vi "RLwithTD.vi"() -> ()   [LabVIEW 2019]
uses:
  <vilib>/Platform/TimedLoop/XDataNode/timing_clust.ctl
  <vilib>/Platform/TimedLoop/XDataNode/nitl_modes.ctl
  <vilib>/Platform/TimedLoop/XDataNode/wakeup.ctl
  <vilib>/Simulation/Shared/_Datatypes/SIM SISO Transfer Function.ctl
  <vilib>/myRIO/Instrument Drivers/Onboard IO/AI/typedefs/AI Reference.ctl
  <vilib>/myRIO/Common/Instrument Driver Framework/Utilities/typedefs/myRIO Generic Hardware Reference.ctl
  <vilib>/myRIO/Common/Instrument Driver Framework/Utilities/typedefs/Hardware Version Enum.ctl
  <vilib>/myRIO/Common/Instrument Driver Framework/Utilities/typedefs/myRIO v1.0 Reference.ctl
  <vilib>/myRIO/Common/Instrument Driver Framework/Utilities/typedefs/Generic FPGA Reference.ctl
  <vilib>/myRIO/Common/Instrument Driver Framework/myRIO v1.0/AI/typedefs/AI Channels List.ctl
  <vilib>/myRIO/Common/Instrument Driver Framework/myRIO v1.0/AI/typedefs/AI Channels Enum.ctl
  <vilib>/myRIO/Common/Instrument Driver Framework/Utilities/typedefs/Analog Scaling Constants List.ctl
  <vilib>/myRIO/Common/Instrument Driver Framework/Utilities/typedefs/Analog Scaling Constants.ctl
  <vilib>/userDefined/High Color/nirio_resource_hc.ctl
  <vilib>/Simulation/Shared/_Datatypes/SIM MIMO State Space.ctl
  <vilib>/myRIO/Instrument Drivers/Onboard IO/AO/typedefs/AO Reference.ctl
  <vilib>/myRIO/Common/Instrument Driver Framework/myRIO v1.0/AO/typedefs/AO Channels List.ctl
  <vilib>/myRIO/Common/Instrument Driver Framework/myRIO v1.0/AO/typedefs/AO Channels Enum.ctl
  <vilib>/myRIO/Common/Instrument Driver Framework/Utilities/vis/Is FPGA Ref Available.vi
  <vilib>/myRIO/Common/Instrument Driver Framework/myRIO v1.0/AI/vis/myRIO v1.1 Open AI.vi
  <vilib>/myRIO/Instrument Drivers/Onboard IO/AI/vis/Read.vi
  <vilib>/Simulation/DiscreteLinear/Implementation/NILVSim Discrete Transfer Function Direct.llb/SIM Discrete Transfer Function Diagram (SISO).vi
  <vilib>/Simulation/DiscreteLinear/Implementation/NILVSim Discrete State Space Direct.llb/SIM Discrete State Space Direct Diagram (SISO).vi
  <vilib>/myRIO/Common/Instrument Driver Framework/myRIO v1.0/AO/vis/myRIO v1.1 Open AO.vi
  <vilib>/myRIO/Instrument Drivers/Onboard IO/AO/vis/Write.vi
  <vilib>/myRIO/Common/Instrument Driver Framework/Utilities/vis/Validate Channels.vi
  <vilib>/myRIO/Common/Instrument Driver Framework/myRIO v1.0/AI/vis/myRIO v1.0 Reserve AI.vi
  <vilib>/Simulation/ContinuousLinear/Implementation/Shared/SIM Transfer Function Support.llb/SIM TransferFunction Normalize to Buffer.vi
  <vilib>/Simulation/DiscreteLinear/Implementation/Shared/SIM Init Discrete States.vi
  <vilib>/Simulation/DiscreteLinear/Implementation/NILVSim Discrete Transfer Function Direct.llb/SIM Transfer Function Direct core (SISO).vi
  <vilib>/Simulation/DiscreteLinear/Implementation/NILVSim Discrete State Space Direct.llb/NILVSim Discrete State Space Direct Diagram Core (SISO).vi
  <vilib>/myRIO/Common/Instrument Driver Framework/myRIO v1.0/AO/vis/myRIO v1.0 Reserve AO.vi
  <vilib>/myRIO/Common/Instrument Driver Framework/myRIO v1.0/AI/vis/myRIO v1.0 Build MUX Configuration AI.vi
  <vilib>/myRIO/Common/Instrument Driver Framework/myRIO v1.0/Resource Manager/vis/myRIO v1.0 Reserve Channel List.vi
  <vilib>/Simulation/ContinuousLinear/Implementation/Shared/SIM Transfer Function Support.llb/SIM TransferFunction Normalize.vi
  <vilib>/myRIO/Common/Instrument Driver Framework/myRIO v1.0/AO/vis/myRIO v1.0 Build MUX Configuration AO.vi
  <vilib>/myRIO/Common/Instrument Driver Framework/myRIO v1.0/Resource Manager/vis/myRIO v1.0 Reserve Channel.vi
  <vilib>/myRIO/Common/Instrument Driver Framework/myRIO v1.0/Resource Manager/vis/myRIO v1.0 Unreserve Channel.vi
  <vilib>/Simulation/Implementation/Shared/SIM Polynomials.llb/SIM Remove Zero Coefficients (DBL).vi
  <vilib>/myRIO/Common/Instrument Driver Framework/myRIO v1.0/Resource Manager/vis/myRIO v1.0 Build Mutex Name.vi
  <vilib>/Simulation/Implementation/Shared/SIM Polynomials.llb/SIM Divide Polynomials (DBL).vi
  <vilib>/Simulation/Implementation/Shared/SIM BuildSimErr.vi
  <vilib>/Utility/VariantDataType/GetNumericInfo.vi
  <vilib>/Utility/error.llb/Error Cluster From Error Code.vi
  <vilib>/myRIO/Common/Instrument Driver Framework/myRIO v1.0/myRIO v1.1 Open.vi
  <vilib>/myRIO/Common/Instrument Driver Framework/myRIO v1.0/AI/vis/myRIO v1.0 Get Scaling Constants AI.vi
  <vilib>/myRIO/Common/Instrument Driver Framework/Utilities/vis/IO Manager.vi
  <vilib>/myRIO/Common/Instrument Driver Framework/Utilities/vis/Configuration Manager.vi
  <vilib>/myRIO/Common/Instrument Driver Framework/myRIO v1.0/myRIO v1.0 Close.vi
  <vilib>/myRIO/Common/Instrument Driver Framework/myRIO v1.0/AI/vis/myRIO v1.0 Read AI.vi
  <vilib>/myRIO/Common/Instrument Driver Framework/myRIO v1.0/AO/vis/myRIO v1.0 Get Scaling Constants AO.vi
  <vilib>/myRIO/Common/Instrument Driver Framework/myRIO v1.0/AO/vis/myRIO v1.0 Write AO.vi
  <vilib>/platform/TimedLoop/XDataNode/XDataNode.xnode
  <vilib>/Simulation/Implementation/XNodeFramework/SimXNode/SimX.xnode
  <vilib>/myRIO/Express VI/Onboard IO/AI/AI Express VI.xnode
  <vilib>/myRIO/Instrument Drivers/Onboard IO/AI/vis/myRIO AI Open.xnode
  <vilib>/myRIO/Express VI/Onboard IO/AO/AO Express VI.xnode
  <vilib>/myRIO/Instrument Drivers/Onboard IO/AO/vis/myRIO AO Open.xnode
  <vilib>/Platform/TimedLoop/XDataNode/XDNodeRunTimeDep.lvlib
  <vilib>/myRIO/Instrument Drivers/Onboard IO/AI/AI.lvlib
  <vilib>/myRIO/Instrument Drivers/Onboard IO/AO/AO.lvlib
  <vilib>/ptbypt/NI_PtbyPt.lvlib
panel:
  out "element":dbl
  in  "Chtter off":bool=TRUE
  in  "psi":dbl=1.0
  in  "Ks":dbl=10.0
  in  "b":dbl=5.0
  in  "hm":dbl=0.01
  in  "Amp step":dbl format="%0.2f"
  in  "D":dbl=16.7
  in  "P":dbl=4689.8
  in  "stopNoise":bool=TRUE
  in  "gain_noise":dbl=0.2
  out "uniform white noise":dbl(graph)=-0.0799803013769669
  in  "AmpWhitehNoise":dbl=1.0 format="%0.2f"
  out "Iteration Duration":i64(graph)=243
  in  "Max FRF current 0-1000mA":dbl=4.0
  in  "Stop FRF":bool=TRUE
  in  "esc":bool
  out "scope":T1(graph)
  out "Current Output EM":dbl(graph)
  in  "Stop EM + FRF":bool=TRUE
  out "left[V]":dbl=-0.0
  out "right[V]":dbl=-0.0
  out "um":dbl=442.3828578
  # "mA"
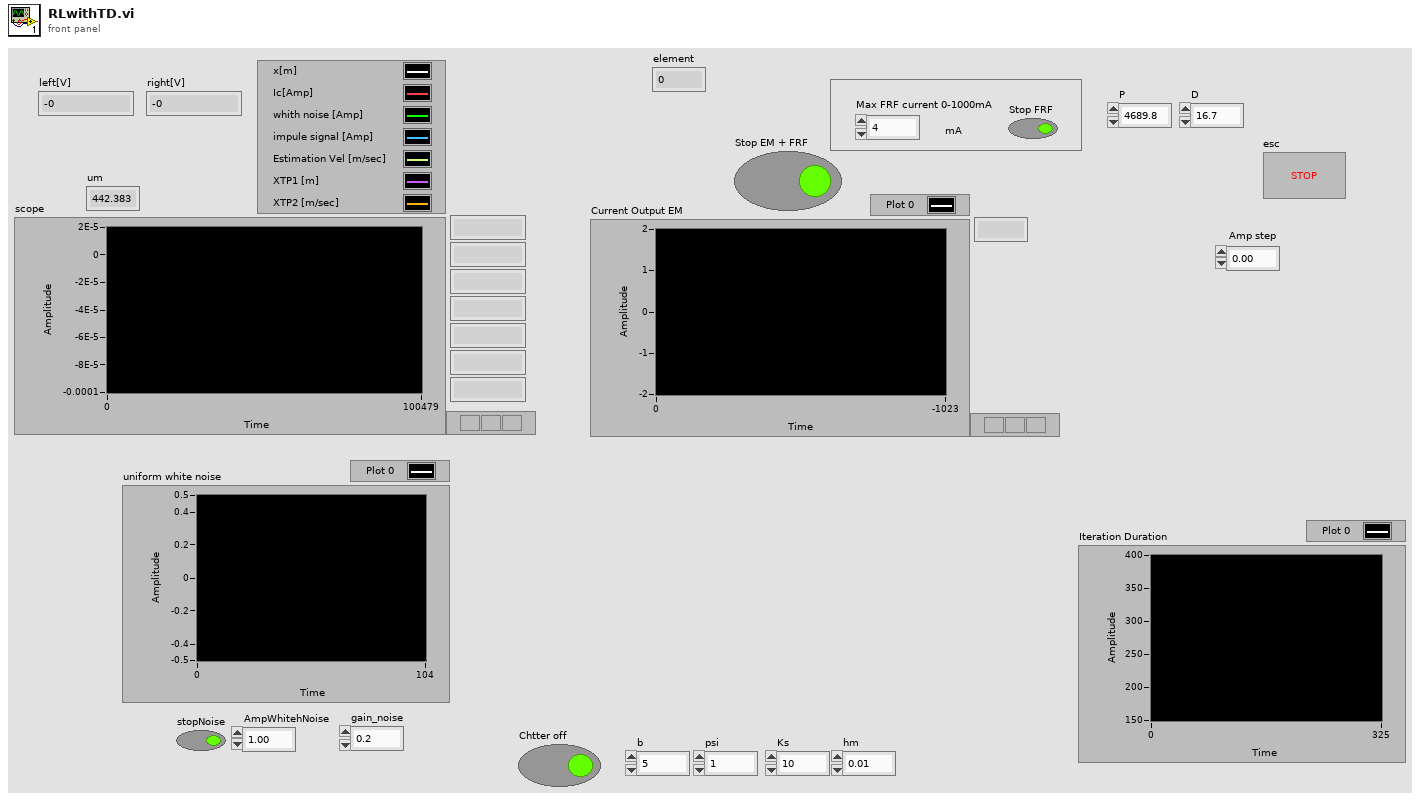
[diagram p1: front panel]
types:
  T1 = cluster{dbl, dbl, dbl, "output y(k)":dbl, dbl, "Numeric":dbl, "Numeric":dbl}
  T2 = typedef "XDNodeRunTimeDep.lvlib/timing_clust.ctl" = cluster{"Expected End [f-1]":u64, "Actual End [f-1]":u64, "Finished Late? [f-1]":bool, "Expected End [i-1]":u64, "Actual End [i-1]":u64, "Finished Late? [i-1]":bool, "Expected Start [i]":u64, "Actual Start [i]":u64, "Expected Start [f]":u64, "Actual Start [f]":u64, "Source Name":string, "Structure Name":string, "Period":i64, "Deadline":i64, "Offset":i64, "Start":i64, "Priority":i32, "Timeout":i32, "Mode":T3, "Wakeup Reason":T4, "Error":errorcluster, "Source Type":string, "Secondary Source Type":string, "Global End Time":u64, "Global Start Time":u64, "Frame Duration":u64, "Iteration Duration":u64, "Assigned CPU":i32, "I/O Scan Engine Mode":u32}
  T3 = typedef "XDNodeRunTimeDep.lvlib/nitl_modes.ctl" = enum32{"No Change", "Process missed periods, maintain original phase", "Discard missed periods, maintain original phase", "Process missed periods, ignore original phase", "Discard missed periods, ignore original phase"}
  T4 = typedef "XDNodeRunTimeDep.lvlib/wakeup.ctl" = enum32{"Normal", "Aborted", "Asynchronous wakeup", "Timing source error", "Timed loop error", "Timeout"}
  T5 = typedef "SIM SISO Transfer Function.ctl" = cluster{"Numerator":dbl[], "Denominator":dbl[]}
  T6 = typedef "SIM MIMO State Space.ctl" = cluster{"A":dbl[][], "B":dbl[][], "C":dbl[][], "D":dbl[][]}
  T7 = typedef "AO.lvlib/AO Reference.ctl" = cluster{"myRIO Reference":T8, "AO Channel List":T12, "AO Scaling Constant List":T14}
  T8 = typedef "myRIO Generic Hardware Reference.ctl" = cluster{"myRIO Model":T9, "myRIO Hardware Reference":T10}
  T9 = typedef "Hardware Version Enum.ctl" = enum16{"Unknown", "myRIO-1900", "myRIO-1950", "roboRIO", "NI ELVIS RIO CM", "ELVIS III"}
  T10 = typedef "myRIO v1.0 Reference.ctl" = cluster{"Generic FPGA Reference":T11, "Allow multiple opens":bool}
  T11 = typedef "Generic FPGA Reference.ctl" = refnum<k20>
  T12 = typedef "AO Channels List.ctl" = T13[]
  T13 = typedef "AO Channels Enum.ctl" = enum16{"Not Connected", "AudioOut/Left", "AudioOut/Right", "C/AO0", "C/AO1", "A/AO0", "A/AO1", "B/AO0", "B/AO1"}
  T14 = typedef "Analog Scaling Constants List.ctl" = T15[]
  T15 = typedef "Analog Scaling Constants.ctl" = cluster{"LSB Weight (Volts)":dbl, "Offset (Volts)":dbl, "Signed?":bool}
  T16 = typedef "nirio_resource_hc.ctl" = tag
  T17 = typedef "AI.lvlib/AI Reference.ctl" = cluster{"myRIO Reference":T8, "AI Channels List":T18, "AI Scaling Constants List":T14}
  T18 = typedef "AI Channels List.ctl" = T19[]
  T19 = typedef "AI Channels Enum.ctl" = enum16{"Not Connected", "AudioIn/Left", "AudioIn/Right", "C/AI0", "C/AI1", "A/AI0", "A/AI1", "A/AI2", "A/AI3", "A/AI4", "A/AI5", "A/AI6", "A/AI7", "B/AI0", "B/AI1", "B/AI2", "B/AI3", "B/AI4", "B/AI5", "B/AI6", "B/AI7", "AI/AI0", "AI/AI1", "AI/AI2", "AI/AI3", "A/AI0 (DIFF)", "A/AI1 (DIFF)", "A/AI2 (DIFF)", "A/AI3 (DIFF)", "B/AI0 (DIFF)", "B/AI1 (DIFF)", "B/AI2 (DIFF)", "B/AI3 (DIFF)"}
  T20 = cluster{dbl, dbl, dbl, dbl, "output y(k)":dbl, "Numeric":dbl, "Numeric":dbl}
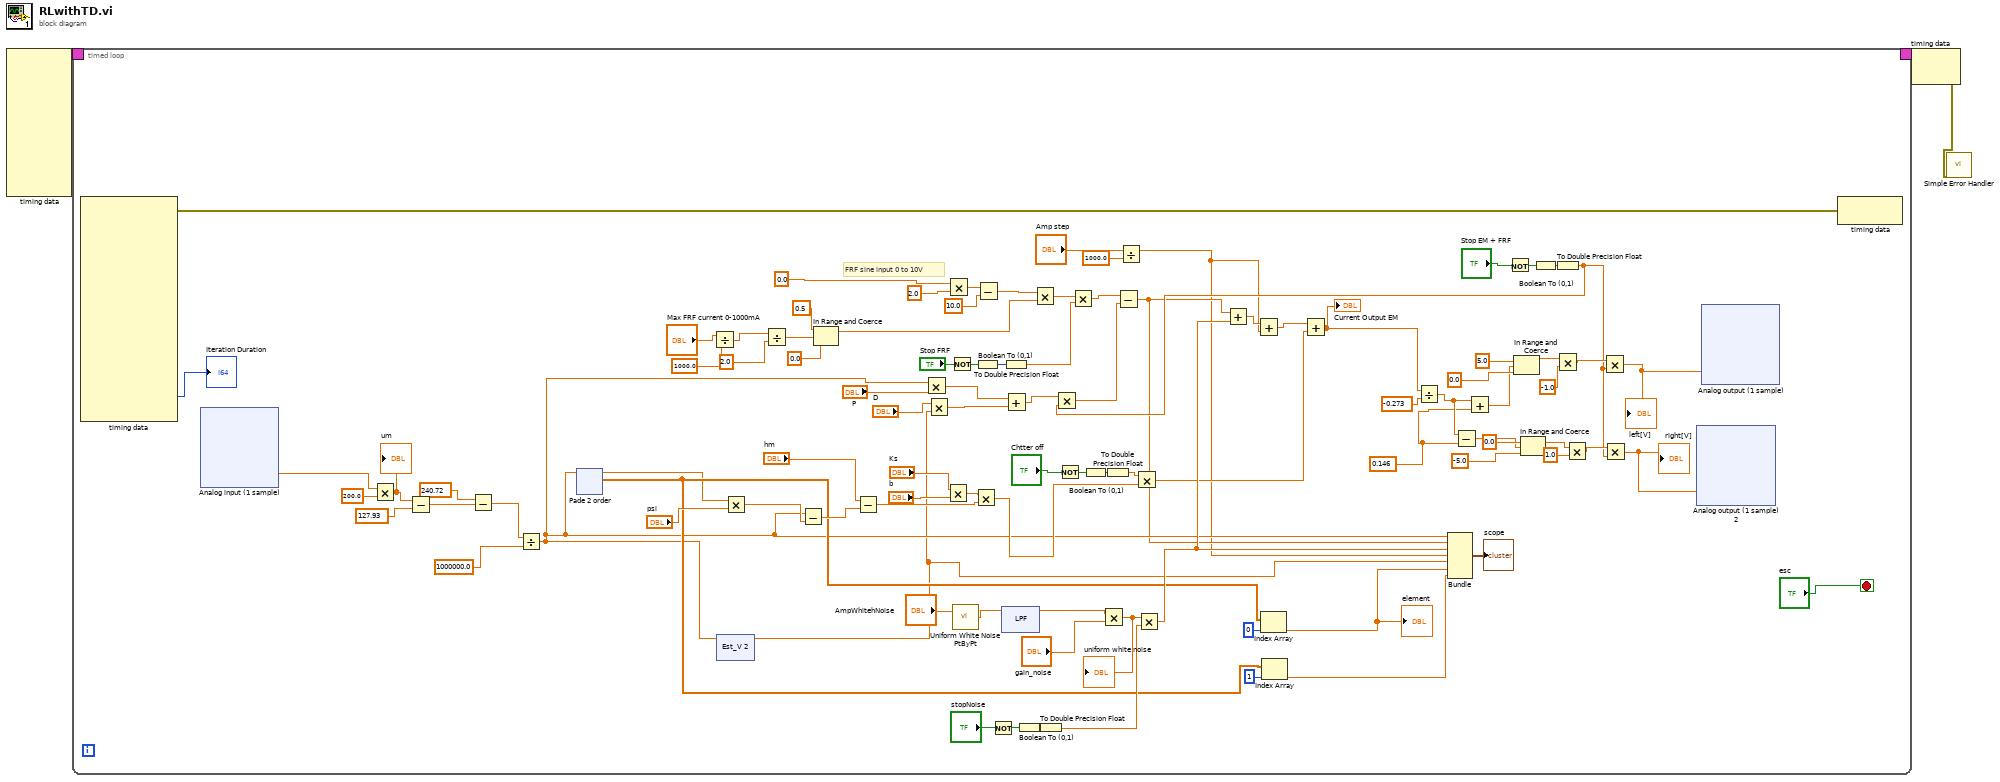
[diagram p0: block diagram]
diagram:
  n1 = node-c288() -> (w3:T2)  [unwired: 10 in]
  n2 = timed-loop {
    timing: w3 -> [_]
    timing-out: [_] -> w2
    stop <- "esc" stop-if-true
    w60 = 0.146 ("y")
    # "FRF sine input 0 to 10V"
    n3 = node-c288() -> (w100:errorcluster, →"Iteration Duration":i64)  [unwired: 1 in, 15 out]
    n4 = xnode "Analog input (1 sample)"() -> ("C/AI1 (AI1)"=w57:dbl)  [unwired: 1 in, 1 out]
    n5 = Multiply(x=w57, y=200.0) -> (x*y=w98:dbl)
    "um" <- w98
    n6 = Subtract(x=w98, y=127.93) -> (x-y=w97:dbl)
    n7 = Subtract(x=240.72, y=w97) -> (x-y=w42:dbl)
    n8 = Divide(x=w42, y=1000000.0) -> (x/y=w8:dbl)
    n9 = xnode "Pade 2 order"("input u(k)"=w8) -> ("state x(k+1)"=w12:dbl[], "output y(k)"=w9:dbl)  [unwired: 2 in, 2 out]
    n10 = Divide(x="Max FRF current 0-1000mA", y=1000.0) -> (x/y=w67:dbl)
    n11 = xnode "Est_V 2"("input u(k)"=w8) -> ("output y(k)"=w7:dbl)  [unwired: 2 in, 1 out]
    n12 = Multiply(x=w9, y="psi") -> (x*y=w18:dbl)
    n13 = Divide(x=w67, y=2.0) -> (x/y=w71:dbl)
    n14 = Subtract(x=w8, y=w18) -> (x-y=w17:dbl)
    n15 = In Range and Coerce(upper limit=0.5, x=w71, lower limit=0.0) -> (coerced(x)=w68:dbl)  [unwired: 1 out]
    n16 = Subtract(x="hm", y=w17) -> (x-y=w32:dbl)
    n17 = Multiply(x=w8, y="P") -> (x*y=w41:dbl)
    n18 = Multiply(x="D", y=w7) -> (x*y=w40:dbl)
    n19 = Multiply(x="Ks", y="b") -> (x*y=w33:dbl)
    n20 = Multiply(x=0.0, y=2.0) -> (x*y=w76:dbl)
    n21 = Not(x="Stop FRF") -> (.not. x?=w80:bool)
    n22 = call <vilib>:"Uniform White Noise PtByPt.vi"("amplitude"="AmpWhitehNoise") -> ("uniform white noise"=w51:dbl)  [unwired: 2 in]
    n23 = Multiply(x=w33, y=w32) -> (x*y=w24:dbl)
    n24 = Boolean To (0,1)(Boolean=w80) -> (0, 1=w79:i16)
    n25 = Subtract(x=w76, y=10.0) -> (x-y=w73:dbl)
    n26 = Not(x="stopNoise") -> (.not. x?=w49:bool)
    n27 = xnode "LPF"("input u(k)"=w51) -> ("output y(k)"=w48:dbl)  [unwired: 2 in, 1 out]
    n28 = To Double Precision Float(number=w79) -> (double precision float=w78:dbl)
    n29 = Add(x=w41, y=w40) -> (x+y=w34:dbl)
    n30 = Boolean To (0,1)(Boolean=w49) -> (0, 1=w50:i16)
    n31 = Multiply(x=w73, y=w68) -> (x*y=w74:dbl)
    n32 = To Double Precision Float(number=w50) -> (double precision float=w45:dbl)
    n33 = Not(x="Chtter off") -> (.not. x?=w26:bool)
    n34 = Multiply(x=w74, y=w78) -> (x*y=w82:dbl)
    n35 = Boolean To (0,1)(Boolean=w26) -> (0, 1=w27:i16)
    n36 = Multiply(x=w48, y="gain_noise") -> (x*y=w44:dbl)
    "uniform white noise" <- w44
    n37 = To Double Precision Float(number=w27) -> (double precision float=w25:dbl)
    n38 = Divide(x="Amp step", y=1000.0) -> (x/y=w5:dbl)
    n39 = Multiply(x=w25, y=w24) -> (x*y=w23:dbl)
    n40 = Multiply(x=w44, y=w45) -> (x*y=w43:dbl)
    n41 = Index Array(array=w12, index=0 ("index (row)")) -> (element=w15:dbl)
    "element" <- w15
    n42 = Index Array(array=w12, index=1) -> (element=w14:dbl)
    n43 = Not(x="Stop EM + FRF") -> (.not. x?=w85:bool)
    n44 = Boolean To (0,1)(Boolean=w85) -> (0, 1=w87:i16)
    n45 = To Double Precision Float(number=w87) -> (double precision float=w35:dbl)
    n46 = Multiply(x=w34, y=w35) -> (x*y=w36:dbl)
    n47 = Subtract(x=w82, y=w36) -> (x-y=w6:dbl)
    n48 = Add(x=w6, y=w43) -> (x+y=w39:dbl)
    n49 = Add(x=w39, y=w5) -> (x+y=w19:dbl)
    n50 = Add(x=w19, y=w23) -> (x+y=w20:dbl)
    "Current Output EM" <- w20
    n51 = Divide(x=w20, y=-0.273) -> (x/y=w61:dbl)
    n52 = Bundle(w8, w6, w43, w5, "output y(k)"=w7, "Numeric"=w15, "Numeric"=w14) -> (→"scope":T20)  [unwired: 1 in]
    n53 = Subtract(x=w61, y=w60) -> (x-y=w62:dbl)
    n54 = Add(x=w61, y=w60) -> (x+y=w63:dbl)
    n55 = In Range and Coerce(upper limit=5.0 ("x"), x=w63, lower limit=0.0) -> (coerced(x)=w54:dbl)  [unwired: 1 out]
    n56 = In Range and Coerce(upper limit=0.0 ("x"), x=w62, lower limit=-5.0) -> (coerced(x)=w90:dbl)  [unwired: 1 out]
    n57 = Multiply(x=w54, y=-1.0) -> (x*y=w59:dbl)
    n58 = Multiply(x=w90, y=1.0) -> (x*y=w58:dbl)
    n59 = Multiply(x=w59, y=w35) -> (x*y=w56:dbl)
    "left[V]" <- w56
    n60 = Multiply(x=w58, y=w35) -> (x*y=w55:dbl)
    "right[V]" <- w55
    n61 = xnode "Analog output (1 sample) 2"("C/AO1 (AO1)"=w55) -> ()  [unwired: 1 in, 1 out]
    n62 = xnode "Analog output (1 sample)"("C/AO0 (AO0)"=w56) -> ()  [unwired: 1 in, 1 out]
    n63 = node-c288(w100) -> ()  [unwired: 1 out]
  }
  n64 = node-c288(w2) -> (w1:errorcluster)
  n65 = call <vilib>:"Simple Error Handler.vi"("error in (no error)"=w1) -> ()  [unwired: 4 in, 5 out]
